vi "Periodic Tasks.vi"(8 "error in":errorcluster) -> ()   [LabVIEW 2015]
doc: "This VI runs in parallel to other tasks. It can contain as many user-defined periodic loops as you need. These can carry out PID or other sorts of timed response."
uses:
  <vilib>/Rock Robotics/WPI/Utilities/WPI_GetSetVariantRefNum.vi
  Robot Global Data.vi
  <vilib>/Rock Robotics/Network Tables/NT Write Number.vi
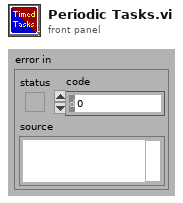
[diagram p1: front panel]
types:
  T1 = typedef "WPI_JoystickDevRef.ctl" = cluster{"Device":T2}
  T2 = typedef "WPI_JoystickDeviceEnum.ctl" = enum16{"USB 0", "USB 1", "USB 2", "USB 3", "USB 4", "USB 5"}
  T3 = typedef "WPI_RobotDriveDevRef.ctl" = cluster{"DevStatus":errorcluster, "Motors[]":T4[], "Square Inputs":bool, "Max Output":dbl}
  T4 = typedef "WPI_MotorControlDeviceRef.ctl" = cluster{"DeviceStatus":errorcluster, "Type":T5, "PWM":cluster{"PWM Channel":T6, "DeadBand":T7}, "CAN":cluster{"Device Number":u8, "Control Mode":T8, "Semaphore":T9, "Max Vout":dbl, "TalonSRX Control Mode":T10}, "Invert":bool}
  T5 = typedef "WPI_MotorControlType.ctl" = enum16{"PWM", "CAN", "CANTalonSRX"}
  T6 = typedef "FPGA_DIOPWMChannel.ctl" = enum8{"PWM 0", "PWM 1", "PWM 2", "PWM 3", "PWM 4", "PWM 5", "PWM 6", "PWM 7", "PWM 8", "PWM 9", "PWM MXP 0", "PWM MXP 1", "PWM MXP 2", "PWM MXP 3", "PWM MXP 4", "PWM MXP 5", "PWM MXP 6", "PWM MXP 7", "PWM MXP 8", "PWM MXP 9", "Invalid"}
  T7 = typedef "WPI_PWMDeadband.ctl" = cluster{"Name":string, "maxPositivePwm":i32, "minPositivePwm":i32, "centerPwm":i32, "maxNegativePwm":i32, "minNegativePwm":i32, "angularRange":u16}
  T8 = typedef "WPI_CANJaguar_ControlMode.ctl" = enum8{"Percent VBus", "Current", "Speed", "Position", "Voltage"}
  T9 = typedef "Semaphore RefNum" = refnum<k1>
  T10 = typedef "WPI_CANTalonSRX_APIControlMode.ctl" = enum8{"Percent VBus", "Speed", "Position", "Slave", "Unchanged / Invalid", "Voltage Compensation", "Current", "Motion Profile"}
  T11 = typedef "WPI_AnalogChannelDevRef.ctl" = cluster{"DevStatus":errorcluster, "Analog Channel":T12}
  T12 = typedef "FPGA_AIChannel.ctl" = enum8{"AI 0", "AI 1", "AI 2", "AI 3", "AI MXP 0", "AI MXP 1", "AI MXP 2", "AI MXP 3", "Invalid"}
  T13 = typedef "WPI_EncoderDevRef.ctl" = cluster{"DevStatus":errorcluster, "EncoderIndex":T14, "CounterIndex":T15, "DistancePerCount":dbl, "Decoding Type":T16}
  T14 = typedef "FPGA_EncoderIdx.ctl" = enum8{"Enc 0", "Enc 1", "Enc 2", "Enc 3", "Enc 4", "Enc 5", "Enc 6", "Enc 7", "Invalid"}
  T15 = typedef "FPGA_CounterCtrSystemIndex.ctl" = enum8{"Ctr 0", "Ctr 1", "Ctr 2", "Ctr 3", "Ctr 4", "Ctr 5", "Ctr 6", "Ctr 7", "Invalid"}
  T16 = typedef "WPI_EncoderType.ctl" = enum16{"1x", "2x", "4x"}
  T17 = typedef "WPI_GyroDevRef.ctl" = cluster{"DevStatus":errorcluster, "Analog Channel":T12, "Offset":dbl, "Gain (VoltsPerDegree/Second)":dbl, "Gyro Type":enum16{"Analog", "XRS450"}, "Handle":i32, "SPI Bus":T18, "Device Found":bool, "Sample Rate":dbl, "Calibrate On Open":bool}
  T18 = typedef "spi_bus.ctl" = enum16{"SPI On-Board, CS0", "SPI On-Board, CS1", "SPI On-Board, CS2", "SPI On-Board, CS3", "SPI MXP", "Invalid"}
  T19 = cluster{"JoystickDevRef":T1, "RobotDriveDevRef":T3}
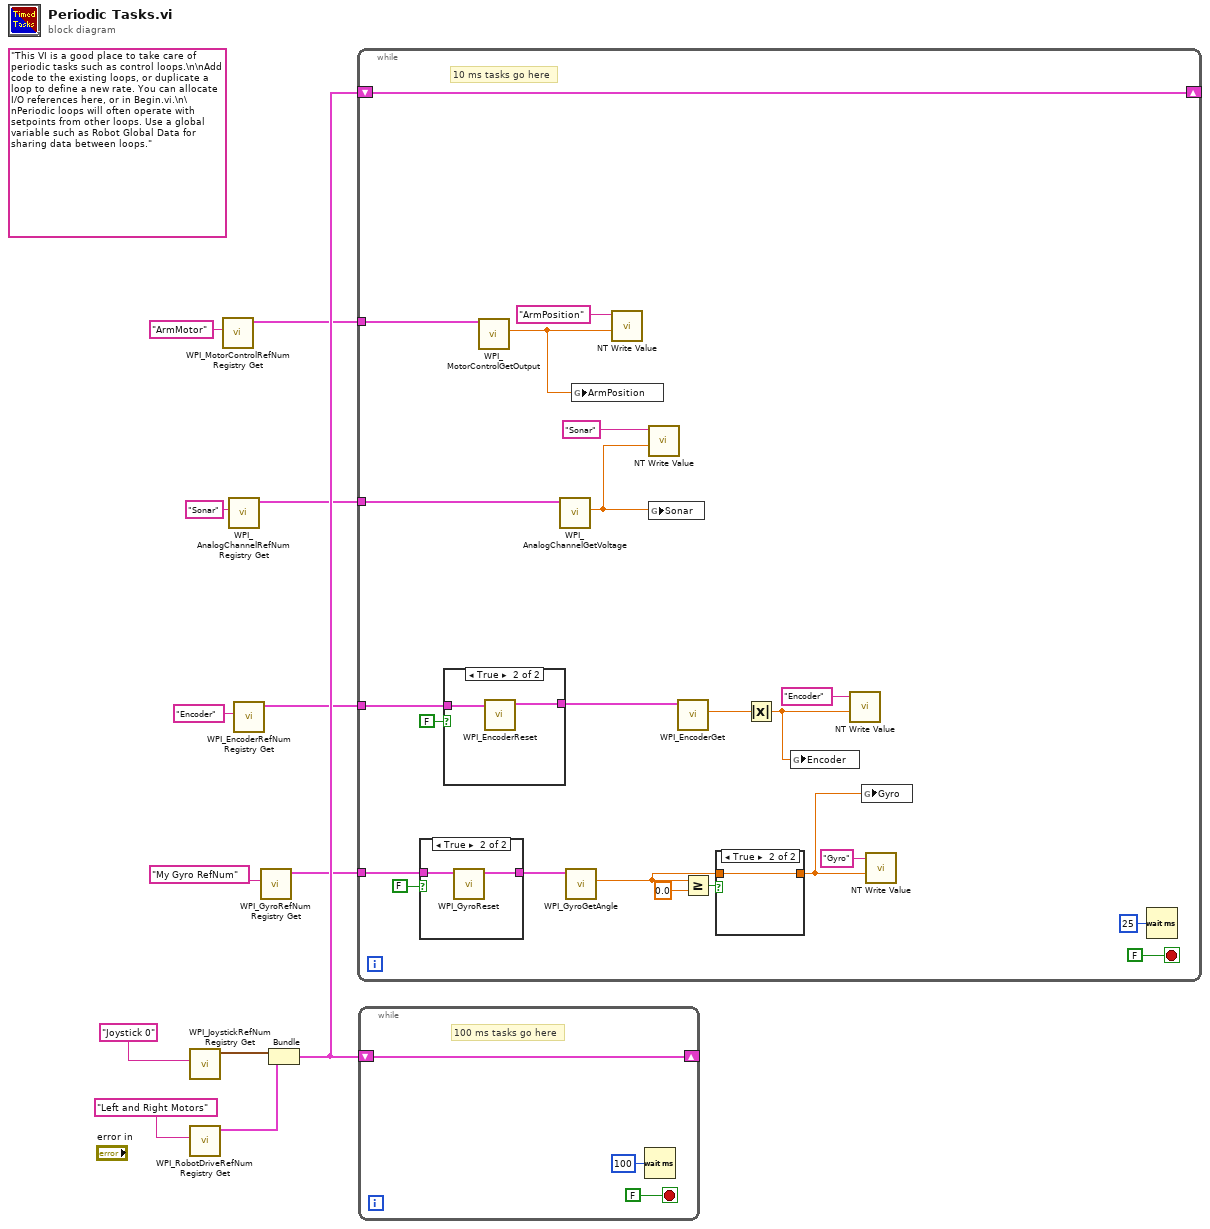
[diagram p0: block diagram]
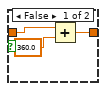
[diagram p3: hidden frame]
diagram:
  (unwired) "This VI is a good place to take care of periodic tasks such as control loops.\n\nAdd code to the existing loops, or duplicate a loop to define a new rate. You can allocate I/O references here, or in Begin.vi.\n\nPeriodic loops will often operate with setpoints from other loops. Use a global variable such as Robot Global Data for sharing data between loops."
  n1 = call <vilib>:"WPI_JoystickRefNum Registry Get.vi"("refnum name"="Joystick 0") -> ("JoystickDevRef"=w11:T1)  [unwired: 1 in, 9 out]
  n2 = call <vilib>:"WPI_RobotDriveRefNum Registry Get.vi"("refnum name"="Left and Right Motors") -> ("RobotDriveDevRef"=w10:T3)  [unwired: 1 in, 9 out]
  n3 = call <vilib>:"WPI_MotorControlRefNum Registry Get.vi"("refnum name"="ArmMotor") -> ("MotorControlDevRef"=w1:T4)  [unwired: 9 in, 1 out]
  n4 = call <vilib>:"WPI_AnalogChannelRefNum Registry Get.vi"("refnum name"="Sonar") -> ("AIDeviceRef"=w3:T11)  [unwired: 9 in, 1 out]
  n5 = call <vilib>:"WPI_EncoderRefNum Registry Get.vi"("refnum name"="Encoder") -> ("EncoderDevRef"=w5:T13)  [unwired: 9 in, 1 out]
  n6 = call <vilib>:"WPI_GyroRefNum Registry Get.vi"("refnum name"="My Gyro RefNum") -> ("GyroDevRef"=w7:T17)  [unwired: 9 in, 1 out]
  n7 = Bundle("JoystickDevRef"=w11, "RobotDriveDevRef"=w10) -> (w9:T19)  [unwired: 1 out]
  n8 = while {
    shift-right: [w34] -> _
    shift-left: w9 -> [w34]
    tunnel: w7 -> [w32]
    tunnel: w5 -> [w25]
    tunnel: w3 -> [w19]
    tunnel: w1 -> [w16]
    stop <- FALSE stop-if-true
    # "10 ms tasks go here"
    n9 = case shown="True" FALSE {
      tunnel: [w44 w45] -> w31
      tunnel: w32 -> [w44 w46]
      frame False {
      }
      frame True {
        n10 = call <vilib>:"WPI_GyroReset.vi"("GyroDevRef"=w46) -> ("GyroDevRef"=w45:T17)  [unwired: 9 in, 1 out]
      }
    }
    n11 = case shown="True" FALSE {
      tunnel: w25 -> [w37 w39]
      tunnel: [w37 w38] -> w23
      frame False {
      }
      frame True {
        n12 = call <vilib>:"WPI_EncoderReset.vi"("EncoderDevRef"=w39) -> ("EncoderDevRef"=w38:T13)  [unwired: 9 in, 1 out]
      }
    }
    n13 = call <vilib>:"WPI_MotorControlGetOutput.vi"("MotorControlDevRef"=w16) -> ("Output"=w14:dbl)  [unwired: 8 in, 2 out]
    n14 = call <vilib>:"WPI_AnalogChannelGetVoltage.vi"("AIDeviceRef"=w19) -> ("Voltage"=w18:dbl)  [unwired: 8 in, 2 out]
    n15 = call <vilib>:"WPI_GyroGetAngle.vi"("GyroDevRef"=w31) -> ("Angle"=w28:dbl)  [unwired: 6 in, 4 out]
    n16 = global write "Robot Global Data.vi" "ArmPosition"(w14) -> ()
    n17 = call-poly <vilib>:"NT Write Value.vi"("Numeric"=w14, "Name"="ArmPosition") -> ()  [unwired: 9 in, 1 out]
    n18 = call-poly <vilib>:"NT Write Value.vi"("Numeric"=w18, "Name"="Sonar") -> ()  [unwired: 9 in, 1 out]
    n19 = global write "Robot Global Data.vi" "Sonar"(w18) -> ()
    n20 = call <vilib>:"WPI_EncoderGet.vi"("EncoderDevRef"=w23) -> ("Distance"=w22:dbl)  [unwired: 5 in, 5 out]
    n21 = Greater Or Equal?(x=w28, y=0.0) -> (x >= y?=w29:bool)
    n22 = case shown="True" w29 {
      tunnel: [w42 w43] -> w26
      tunnel: w28 -> [w41 w43]
      frame False {
        n23 = Add(x=w41, y=360.0) -> (x+y=w42:dbl)
      }
      frame True {
      }
    }
    n24 = Absolute Value(x=w22) -> (abs(x)=w20:dbl)
    n25 = global write "Robot Global Data.vi" "Encoder"(w20) -> ()
    n26 = call-poly <vilib>:"NT Write Value.vi"("Numeric"=w20, "Name"="Encoder") -> ()  [unwired: 9 in, 1 out]
    n27 = global write "Robot Global Data.vi" "Gyro"(w26) -> ()
    n28 = call-poly <vilib>:"NT Write Value.vi"("Numeric"=w26, "Name"="Gyro") -> ()  [unwired: 9 in, 1 out]
    n29 = Wait (ms)(milliseconds to wait=u32 25) -> ()  [unwired: 1 out]
  }
  n30 = while {
    shift-right: [w47] -> _
    shift-left: w9 -> [w47]
    stop <- FALSE stop-if-true
    # "100 ms tasks go here"
    n31 = Wait (ms)(milliseconds to wait=u32 100) -> ()  [unwired: 1 out]
  }
